vi "Add Prefix.vi"(8 "error in (no error)":errorcluster, 10 "Prefix":string, 11 "Parent in":refnum<class "Parent.lvclass">) -> (0 "error out":errorcluster, 2 "Concatenated String":string, 3 "Parent out":refnum<class "Parent.lvclass">)   [LabVIEW 2023, in "Parent.lvclass"]
doc: "This is a member VI of Parent.lvclass, which contains an input and an output of the LabVIEW class data type . Use this VI as the VI under test for the Add Prefix test in this example."
uses:
  Parent.lvclass
  Parent.lvclass/Parent.ctl
panel:
  # "Overview: This is a member VI of Parent. lvclass, which contains an input and an output of the LabVIEW class data type.\nRequirements: LabVIEW Full Development System, Unit Test Framework Toolkit\nInstructions:\n1.  In the Project Explorer window, right-click Result and select Unit Tests>>Run from the shortcut menu.\n2. \tView the test results in the Unit Test Framework Results windows.\n3. \tIn the Project Explorer window, double-click Add Prefix.lvtest to display the Test Properties dialog box. Read the comments on the Test Cases page to understand why this test passes.\n4.\t In the Test Properties dialog box, you cannot edit the Parent in input and Parent out output because they are of the LabVIEW class data type. However, you can configure the input and expected values by using the front panel of the VI under test, setup VI, and teardown VI, accessible by clicking the Export Values to VI button, and then clicking the Import Values from VI to import the updated values to the current test case."
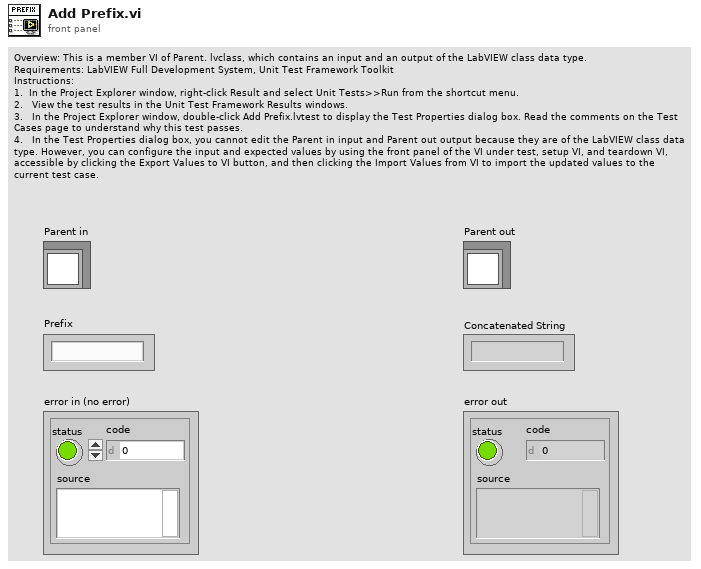
[diagram p1: front panel]
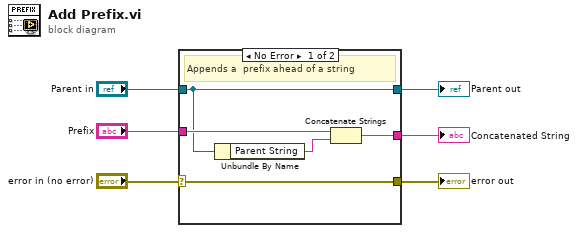
[diagram p0: block diagram]
diagram:
  n1 = case shown="No Error" "error in (no error)" {
    selector: "error in (no error)" -> [w11 w13]
    tunnel: [w11 w13] -> w5
    tunnel: [w7 w12] -> w3
    tunnel: "Parent in" -> [w7 w12]
    tunnel: "Prefix" -> [w10 _]
    tunnel: [w8 _] -> w1
    frame No Error {
      # "Appends a  prefix ahead of a string"
      n2 = Unbundle By Name(w7) -> ("Parent String"=w9:string)
      n3 = Concatenate Strings(w10, w9) -> (w8:string)
    }
    frame Error {
    }
  }
  "error out" <- w5
  "Parent out" <- w3
  "Concatenated String" <- w1
